vi "VI PMA Konfig.vi"() -> ()   [LabVIEW 2020, in "ABB-EL3000.lvlib" / "PMA.lvlib"]
uses:
  PMA.lvlib
  Visualisierungs Elemente/Zahlen-Ausgabefeld.ctl
  CalGas Aufschaltung/Aufschaltung CalGas_ANZEIGE.ctl
  Visualisierungs Elemente/Auswahlfeld.ctl
  FT-IR/FGV FT-IR Gasliste Aktionen.ctl
  Aktion PMA Daten allgemein.ctl
  CalGas Aufschaltung/FGV CalGas Aktionen.ctl
  Messdaten/Aktionen FGV Messdaten.ctl
  Aktion FGV Messwerte.ctl
  Passwortverwaltung/FGV Passwort Aktion.ctl
  Analysator Definition/FGV Analysator Definition Aktionen.ctl
  Kalibrieren/Kalibrierung O2.ctl
  FT-IR/FGV FT-IR Parameter.vi
  Messdaten/Messdaten.lvlib
  Passwortverwaltung/Passwort.lvlib
  Analysator Definition/Analysator Definition.lvlib
  FT-IR/FT-IR.lvlib
  Allgemein/allgemeine Sub-VIs.lvlib
  Allgemeine VI/Allgemeine VI.lvlib
  Kalibrieren/Kalibrieren.lvlib
  Allgemeine VI/Aktionen Cal Daten speichern.ctl
  CalGas Aufschaltung/CalGas Aufschaltung.lvlib
  Grafik/Grafik.lvlib
panel:
  out "Kal. Wert O2:":T1 caption="Konzentration" format="%.3f"
  out "Roh Wert O2:":sgl format="%.3f"
  in  "Kalidaten":bool
  in  "Calibration with Ambient Air:":bool
  in  "Automatic Concentration:":sgl caption="%" format="%#_5g"
  in  "Manuel Concentration:":sgl caption="%" format="%#_5g"
  in  "Calibration Mode:":enum16{"Manuel", "Automatic"}(ring)
  in  "Endpunkt":bool
  in  "0-Punkt":bool
  in  "O2 Messbereich":u16(ring)
  out "Wartungsbedarf":bool
  out "Funktionskontrolle":bool
  out "Ausfall":bool
  out "Druck Detektor:":sgl format="%#.1f"
  out "Temperatur Regler:":sgl format="%#.1f"
  out "Stellgröße Regler":sgl caption="%" format="%#.1f"
  out "Temperatur Detektor:":sgl format="%#.1f"
  out "Mwert":sgl format="%.3f"
  out "PMwert":sgl format="%.3f"
  out "O2":string
  out "Wert":T1 caption="Konzentration" format="%.3f"
  out "Graph1":waveform(dbl)[](graph)
  in  "Aufschaltung CalGas":T2 {"Aufschaltpunkt" items=["Filterblock", "Analysator direkt", "PNS", "Entnahme", "Gasdivider"]; "Kalibriergas" items=["Stickstoff"]}
  # "Konfiguration PMD"
  # "PMD"
  # "Hilfsgrößen:"
  # "Temperatur:"
  # "Stellgröße:"
  # "°C"
  # "°C"
  # "Druck:"
  # "hPa"
  # "STATUS"
  # "Aufschaltung Kalibriergas"
  # "Kalibriergas"
  # "Aufschaltpunkt"
  # "Analysator"
  # "Calibration Parameters"
  # "%"
  # "%"
  # "±"
  # "x"
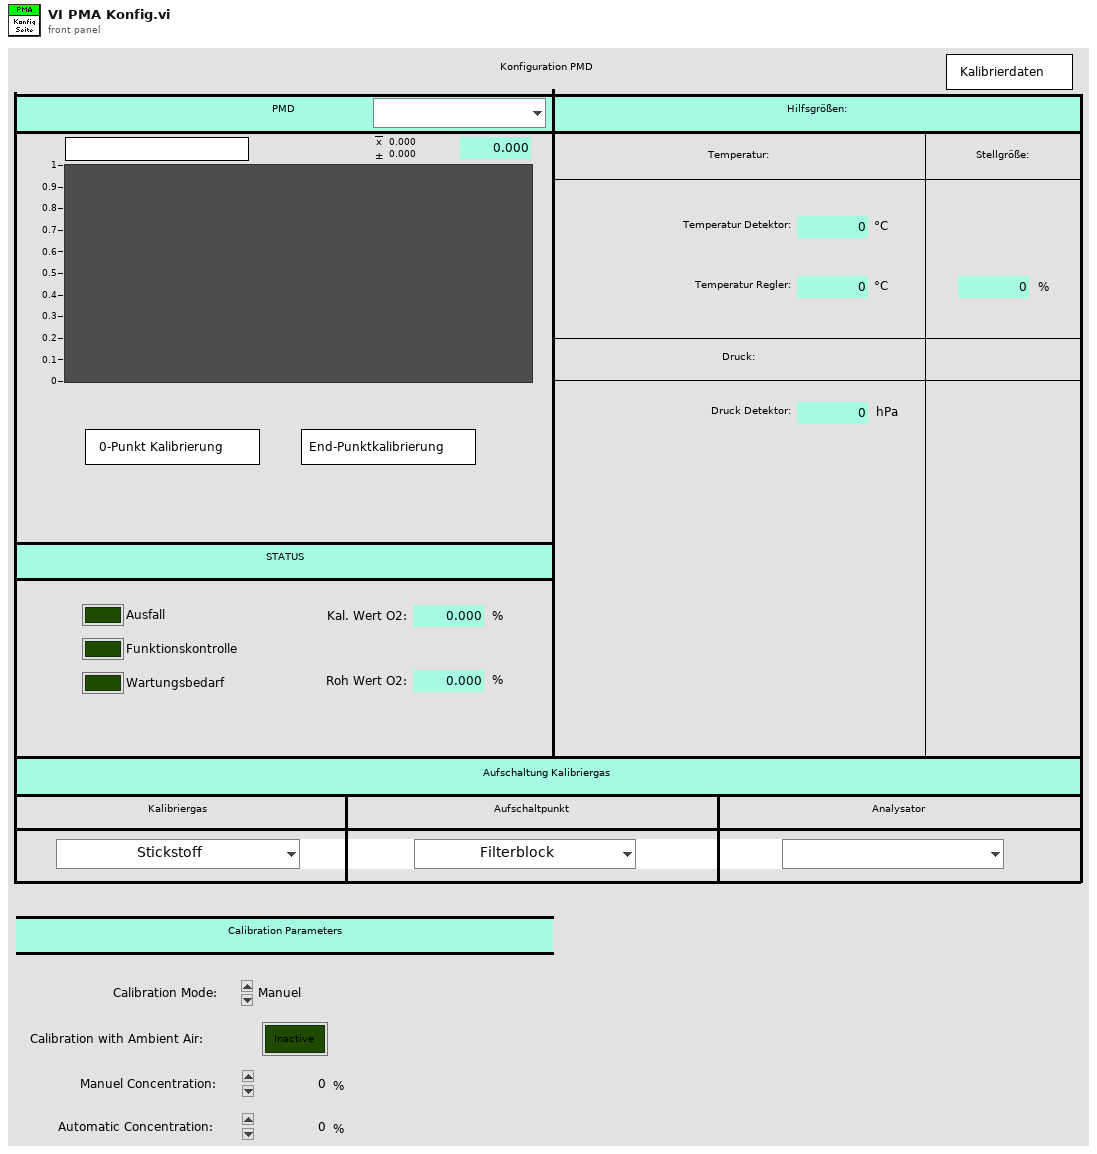
[diagram p1: front panel]
types:
  T1 = typedef "Zahlen-Ausgabefeld.ctl" = sgl
  T2 = typedef "CalGas Aufschaltung.lvlib/Aufschaltung CalGas_ANZEIGE.ctl" = cluster{"Kalibriergas":T3, "Aufschaltpunkt":T3, "Analysator":T3}
  T3 = typedef "Auswahlfeld.ctl" = u16
  T4 = typedef "CalGas Aufschaltung.lvlib/FGV CalGas Aktionen.ctl" = enum16{"lesen", "Analysator Auswahl", "Def.CalGas", "Aufschaltung CalGas", "laden", "speichern", "KAL extrahieren"}
  T5 = typedef "ABB-EL3000.lvlib/PMA.lvlib/Aktion PMA Daten allgemein.ctl" = enum16{"lesen", "schreiben", "laden ", "speichern"}
  T6 = typedef "FT-IR.lvlib/FGV FT-IR Gasliste Aktionen.ctl" = enum16{"lesen", "Gasliste FT-IR", "Gasliste ausgelesen", "laden", "speichern", "löschen"}
  T7 = typedef "ABB-EL3000.lvlib/PMA.lvlib/PMA Daten allgemein.ctl" = cluster{"Autokal aktiv":enum16{"Manuel", "Automatic"}, "Umgebungsluft Kalibration":bool}
  T8 = typedef "String - Ausgabefeld.ctl" = string
  T9 = typedef "CalGas Aufschaltung.lvlib/Aufschaltung CalGas.ctl" = cluster{"Kalibriergas":T3, "Aufschaltpunkt":T10, "Analysator":T11}
  T10 = typedef "CalGas Aufschaltung.lvlib/Auswahl Aufschaltpunkt.ctl" = enum16{"über Filterblock", "Analysator direkt", "über PNS", "Entnahme", "Gasdivider"}
  T11 = typedef "CalGas Aufschaltung.lvlib/Auswahl Analysator.ctl" = enum16{"FT-IR", "FID", "PMA", "PMA/FID/FT-IR"}
  T12 = typedef "CalGas Aufschaltung.lvlib/Definition CalGas Anzeige.ctl" = cluster{"Namen":T13, "Werte":T15, "Werte 2":T15, "Einheit":T17, "Messbereiche":T18}
  T13 = typedef "CalGas Aufschaltung.lvlib/CalGas-Namen.ctl" = cluster{"Name":T14, "Name 2":T14, "Name 3":T14, "Name 4":T14, "Name 5":T14, "Name 6":T14, "Name 7":T14, "Name 8":T14, "Name 9":T14, "Name 10":T14, "Name 11":T14, "Name 12":T14}
  T14 = typedef "String - Eingabefeld.ctl" = string
  T15 = typedef "CalGas Aufschaltung.lvlib/CalGas-Werte.ctl" = cluster{"Konzentration 1":T16, "Konzentration 2":T16, "Konzentration 3":T16, "Konzentration 4":T16, "Konzentration 5":T16, "Konzentration 6":T16, "Konzentration 7":T16, "Konzentration 8":T16, "Konzentration 9":T16, "Konzentration 10":T16, "Konzentration 11":T16, "Konzentration 12":T16}
  T16 = typedef "Zahlen-Eingabefeld.ctl" = sgl
  T17 = typedef "CalGas Aufschaltung.lvlib/CalGas-Einheit.ctl" = cluster{"Einheit 1":T3, "Einheit 2":T3, "Einheit 3":T3, "Einheit 4":T3, "Einheit 5":T3, "Einheit 6":T3, "Einheit 7":T3, "Einheit 8":T3, "Einheit 9":T3, "Einheit 10":T3, "Einheit 11":T3, "Einheit 12":T3}
  T18 = typedef "CalGas Aufschaltung.lvlib/CalGas-Messbereiche.ctl" = cluster{"Messbereich 1":T3, "Messbereich 2":T3, "Messbereich 3":T3, "Messbereich 4":T3, "Messbereich 5":T3, "Messbereich 6":T3, "Messbereich 7":T3, "Messbereich 8":T3, "Messbereich 9":T3, "Messbereich 10":T3, "Messbereich 11":T3, "Messbereich 12":T3}
  T19 = typedef "ABB-EL3000.lvlib/PMA.lvlib/Aktion FGV Messwerte.ctl" = enum16{"lesen", "Messwerte", "Messbereich", "Status", "Diagnose Werte"}
  T20 = typedef "Messdaten.lvlib/Aktionen FGV Messdaten.ctl" = enum16{"lesen", "schreiben", "löschen", "Mittelwerte", "Komponente"}
  T21 = typedef "ABB-EL3000.lvlib/Allgemeine VI.lvlib/Aktionen Cal Daten speichern.ctl" = enum16{"Cal Daten", "Toleranzen", "PMA", "FID", "Cal Daten PMA", "Cal Daten FID"}
  T22 = typedef "Passwort.lvlib/FGV Passwort Aktion.ctl" = enum16{"prüfen", "setzen", "Initialisieren", "PW speichern", "lesen", "PW Änderung"}
  T23 = typedef "Analysator Definition.lvlib/FGV Analysator Definition Aktionen.ctl" = enum16{"lesen", "MB setzen", "MB KAL setzen", "laden"}
  T24 = typedef "ABB-EL3000.lvlib/PMA.lvlib/Kalibrieren.lvlib/Kalibrierung O2.ctl" = enum16{"Nullpunkt O2", "Endpunkt O2"}
  T25 = cluster{"Temp. Detektor":sgl, "Temp. Regler":sgl, "STG Regler":sgl, "Druck Detektor":sgl}
  T26 = cluster{"Ausfall":bool, "Funktionskontrolle":bool, "Wartungsbedarf":bool}
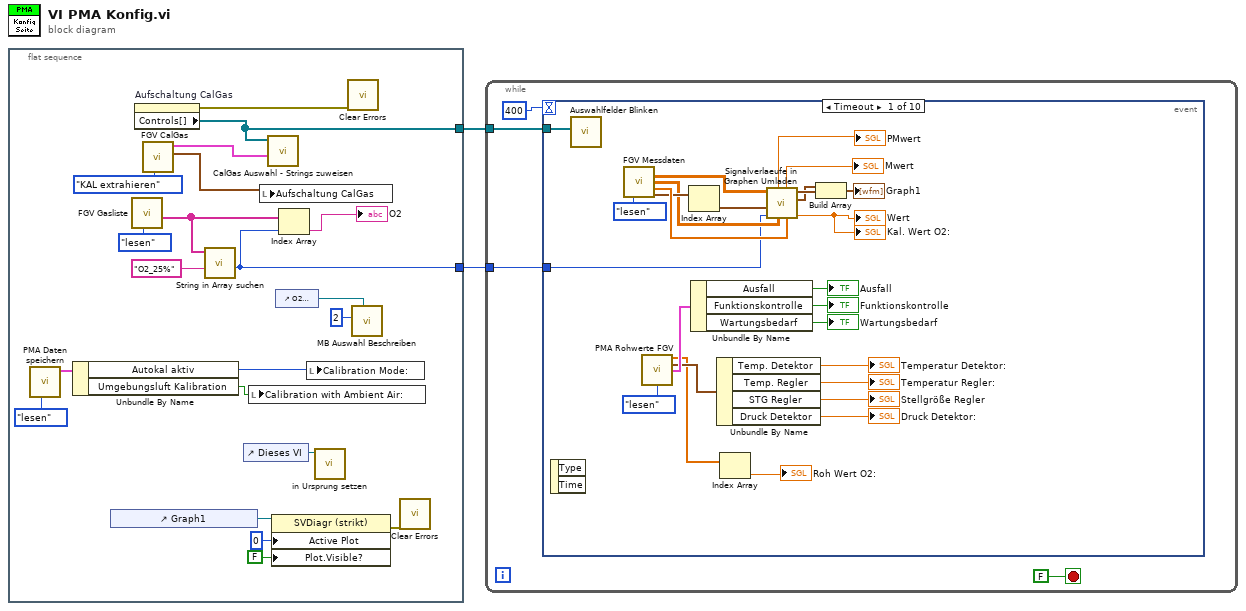
[diagram p0: block diagram]
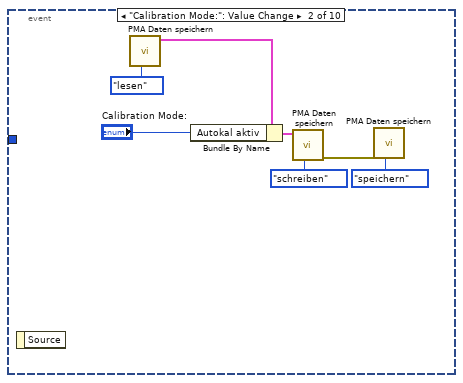
[diagram p2: hidden frame]
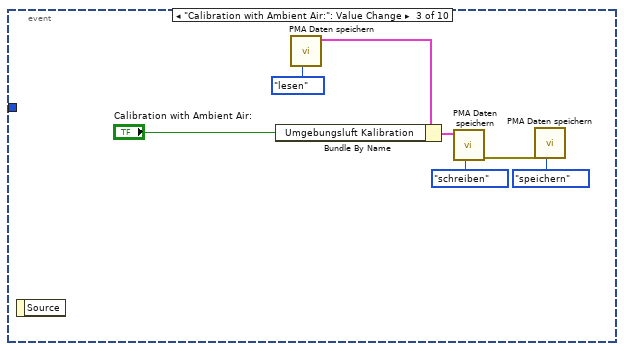
[diagram p3: hidden frame]
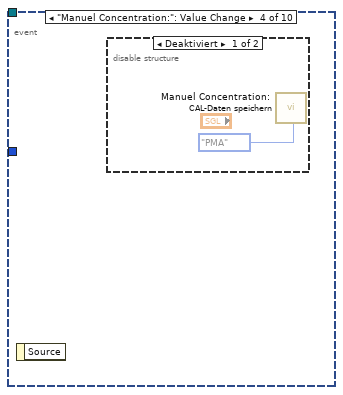
[diagram p4: hidden frame]
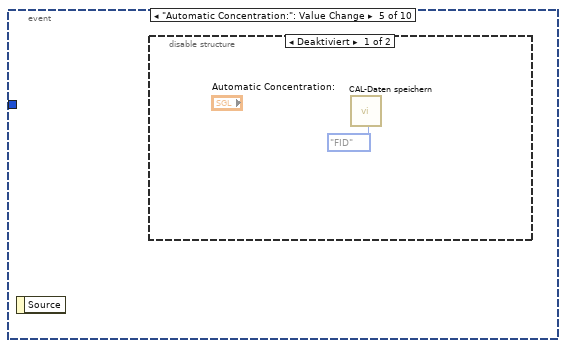
[diagram p6: hidden frame]
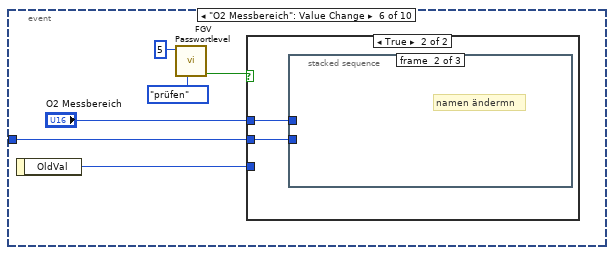
[diagram p8: hidden frame]
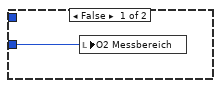
[diagram p9: hidden frame]
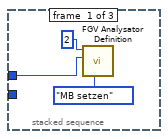
[diagram p10: hidden frame]
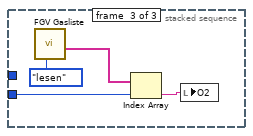
[diagram p11: hidden frame]
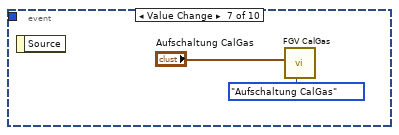
[diagram p12: hidden frame]
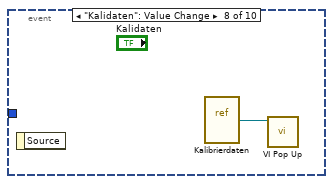
[diagram p13: hidden frame]
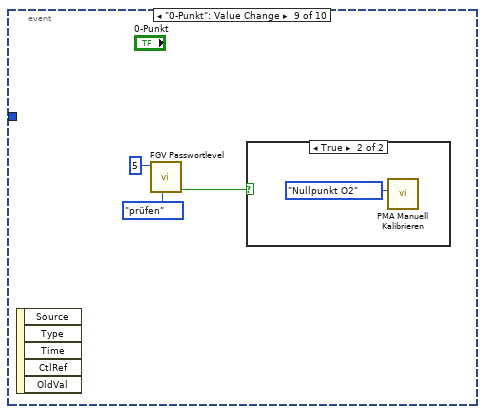
[diagram p14: hidden frame]
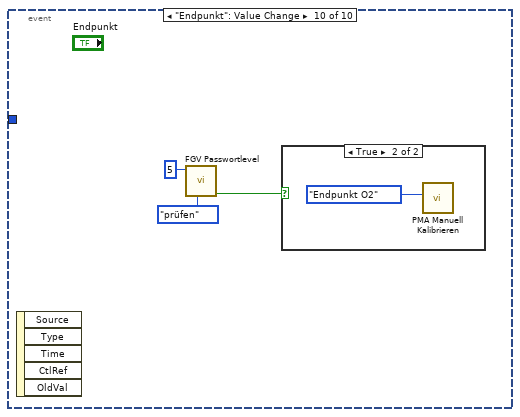
[diagram p16: hidden frame]
diagram:
  n1 = flat-sequence {
    tunnel: [w19] -> w2
    tunnel: [w3] -> w1
    frame #0 {
      n2 = call "PMA Daten speichern.vi"("Aktion"=Aktion_PMA_Daten_allgemein."lesen") -> ("PMA Daten allgemein"=w10:T7)  [unwired: 9 in, 1 out]
      n3 = Unbundle By Name(w10) -> ("Autokal aktiv"=w9:enum16{"Manuel", "Automatic"}, "Umgebungsluft Kalibration"=w8:bool)
      n4 = control-ref of="Graph1"() -> (w15:refnum<vi>)
      n5 = call "FGV Gasliste.vi"("Aktionen"=FGV_FT-IR_Gasliste_Aktionen."lesen") -> ("Aktuelle Gasliste gesamt"=w21:T8[])  [unwired: 8 in, 2 out]
      n6 = property on="Aufschaltung CalGas" class="Cluster (strikt)"() -> (error out=w4:errorcluster, "Controls[]"=w3:refnum<vi>[])  [unwired: 2 in, 1 out]
      n7 = call "FGV CalGas.vi"("Aktionen"=FGV_CalGas_Aktionen."KAL extrahieren") -> ("Aufschaltung CalGas"=w6:T9, "Def.CalGas"=w5:T12)  [unwired: 6 in, 3 out]
      n8 = call "String in Array suchen.vi"("Nach String/Zeichen suchen (-)"="O2_25%" ("DataSocket:URL"), "String-Array"=w21) -> ("Index"=w19:i32)  [unwired: 7 in, 2 out]
      n9 = control-ref of="Dieses VI"() -> (w20:refnum<vi>)
      n10 = local write "Calibration with Ambient Air:"(w8) -> ()
      n11 = local write "Aufschaltung CalGas"(w6) -> ()
      n12 = call "CalGas Auswahl - Strings zuweisen.vi"("Def.CalGas"=w5, "Aufschaltung CalGas"=w3) -> ()  [unwired: 9 in, 1 out]
      n13 = property class="SVDiagr (strikt)"(reference=w15, "Active Plot"=u32 0 ("Aktiver Plot"), "Plot.Visible?"=FALSE ("Plot.Sichtbar")) -> (error out=w12:errorcluster)  [unwired: 1 in, 1 out]
      n14 = control-ref of="O2 Messbereich"() -> (w17:refnum<vi>)
      n15 = Index Array(array=w21, index=w19) -> (element=→"O2":T8)
      n16 = local write "Calibration Mode:"(w9) -> ()
      n17 = call "in Ursprung setzen.vi"("VI Referenz"=w20) -> ()  [unwired: 10 in, 1 out]
      n18 = call <vilib>:"Clear Errors.vi"("error in (no error)"=w4) -> ()  [unwired: 5 in, 2 out]
      n19 = call "MB Auswahl Beschreiben.vi"("Auswahl Referenz"=w17, "Komponente"=2) -> ()  [unwired: 10 in]
      n20 = call <vilib>:"Clear Errors.vi"("error in (no error)"=w12) -> ()  [unwired: 5 in, 2 out]
    }
  }
  n21 = while {
    tunnel: w2 -> [w25]
    tunnel: w1 -> [w24]
    stop <- FALSE stop-if-true
    n22 = event shown="[0] Timeout" {
      selector: _ -> [_ _ _ _ _ _ _ _ _ _]
      dyn-events: _ -> [_ _ _ _ _ _ _ _ _ _]
      timeout: 400 -> [_ _ _ _ _ _ _ _ _ _]
      tunnel: w25 -> [w36 _ _ _ _ w71 _ _ _ _]
      tunnel: w24 -> [w30 _ _ _ _ _ _ _ _ _]
      event Timeout {
        n23 = event-data() -> ()  [unwired: 1 in, 2 out]
        n24 = call "Auswahlfelder Blinken.vi"("Controls[]"=w30) -> ()  [unwired: 11 in]
        n25 = call "FGV Messdaten.vi"("Aktionen"=Aktionen_FGV_Messdaten."lesen") -> ("Messdaten"=w49:sgl[][], "Mittelwertdaten"=w48:sgl[][], "Deviation"=w53:sgl[], "Zeitstempeln"=w51:timestamp[])  [unwired: 6 in, 5 out]
        n26 = call "PMA Rohwerte FGV.vi"("Aktion"=Aktion_FGV_Messwerte."lesen") -> ("Messwerte"=w32:sgl[], "Diagnose Werte"=w40:T25, "Status"=w44:T26)  [unwired: 11 in, 1 out]
        n27 = Index Array(array=w51) -> (element=w52:timestamp)  [unwired: 1 in]
        n28 = Unbundle By Name(w44) -> ("Ausfall"=→"Ausfall":bool, "Funktionskontrolle"=→"Funktionskontrolle":bool, "Wartungsbedarf"=→"Wartungsbedarf":bool)
        n29 = Unbundle By Name(w40) -> ("Temp. Detektor"=→"Temperatur Detektor:":sgl, "Temp. Regler"=→"Temperatur Regler:":sgl, "STG Regler"=→"Stellgröße Regler":sgl, "Druck Detektor"=→"Druck Detektor:":sgl)
        n30 = Index Array(array=w32) -> (element=→"Roh Wert O2:":sgl)  [unwired: 1 in]
        n31 = call "Signalverlaeufe in Graphen Umladen.vi"("Deviation"=w53, "Mittelwertdaten"=w48, "Gas-Auswahl"=w36, "t0"=w52, "Werte"=w49) -> ("Konzentration"=→"Wert" →"Kal. Wert O2:":sgl, "Mittelwert"=w34:waveform(dbl), "Waveform"=w35:waveform(dbl), "aktuelle Mittelwert"=→"Mwert":sgl, "Deviation"=→"PMwert":sgl)  [unwired: 2 in]
        n32 = Build Array(w34, w35) -> (→"Graph1":waveform(dbl)[])
      }
      event "Calibration Mode:": Value Change {
        n33 = event-data() -> ()  [unwired: 1 in, 1 out]
        n34 = call "PMA Daten speichern.vi"("Aktion"=Aktion_PMA_Daten_allgemein."lesen") -> ("PMA Daten allgemein"=w56:T7)  [unwired: 9 in, 1 out]
        n35 = Bundle By Name(cluster=w56, "Autokal aktiv"="Calibration Mode:") -> (w55:T7)
        n36 = call "PMA Daten speichern.vi"("Aktion"=Aktion_PMA_Daten_allgemein."schreiben", "PMA Daten allgemein"=w55) -> ("error out"=w58:errorcluster)  [unwired: 8 in, 1 out]
        n37 = call "PMA Daten speichern.vi"("Aktion"=Aktion_PMA_Daten_allgemein."speichern", "error in (no error)"=w58) -> ()  [unwired: 8 in, 2 out]
      }
      event "Calibration with Ambient Air:": Value Change {
        n38 = event-data() -> ()  [unwired: 1 in, 1 out]
        n39 = call "PMA Daten speichern.vi"("Aktion"=Aktion_PMA_Daten_allgemein."lesen") -> ("PMA Daten allgemein"=w63:T7)  [unwired: 9 in, 1 out]
        n40 = Bundle By Name(cluster=w63, "Umgebungsluft Kalibration"="Calibration with Ambient Air:") -> (w62:T7)
        n41 = call "PMA Daten speichern.vi"("Aktion"=Aktion_PMA_Daten_allgemein."schreiben", "PMA Daten allgemein"=w62) -> ("error out"=w65:errorcluster)  [unwired: 8 in, 1 out]
        n42 = call "PMA Daten speichern.vi"("Aktion"=Aktion_PMA_Daten_allgemein."speichern", "error in (no error)"=w65) -> ()  [unwired: 8 in, 2 out]
      }
      event "Manuel Concentration:": Value Change {
        n43 = event-data() -> ()  [unwired: 1 in, 1 out]
        n44 = disable-structure shown="Deaktiviert" {
          frame Disabled {
            n45 = call "CAL-Daten speichern.vi"("Aktionen Kal Daten speichern"=Aktionen_Cal_Daten_speichern."PMA") -> ()  [unwired: 19 in]
          }
          frame Enabled {
          }
        }
      }
      event "Automatic Concentration:": Value Change {
        n46 = event-data() -> ()  [unwired: 1 in, 1 out]
        n47 = disable-structure shown="Deaktiviert" {
          frame Disabled {
            n48 = call "CAL-Daten speichern.vi"("Aktionen Kal Daten speichern"=Aktionen_Cal_Daten_speichern."FID") -> ()  [unwired: 19 in]
          }
          frame Enabled {
          }
        }
      }
      event "O2 Messbereich": Value Change {
        n49 = event-data() -> ("OldVal"=w72:u16)  [unwired: 1 in]
        n50 = call "FGV Passwortlevel.vi"("FGV Passwort Aktion"=FGV_Passwort_Aktion."prüfen", "geforderter Level"=i16 5) -> ("Freigabe"=w73:bool)  [unwired: 7 in, 2 out]
        n51 = case shown="True" w73 {
          tunnel: w72 -> [w76 _]
          tunnel: w71 -> [_ w78]
          tunnel: "O2 Messbereich" -> [_ w77]
          frame False {
            n52 = local write "O2 Messbereich"(w76) -> ()
          }
          frame True {
            n53 = stacked-sequence {
              tunnel: w78 -> [_ _ w83]
              tunnel: w77 -> [w79 _ _]
              frame #0 {
                n54 = call "FGV Analysator Definition.vi"("Aktionen"=FGV_Analysator_Definition_Aktionen."MB setzen", "Messbereich"=w79, "Komponente"=2) -> ()  [unwired: 4 in, 5 out]
              }
              frame #1 {
                # "namen ändermn"
              }
              frame #2 {
                n55 = call "FGV Gasliste.vi"("Aktionen"=FGV_FT-IR_Gasliste_Aktionen."lesen") -> ("Aktuelle Gasliste gesamt"=w85:T8[])  [unwired: 8 in, 2 out]
                n56 = Index Array(array=w85, index=w83) -> (element=w82:T8)
                n57 = local write "O2"(w82) -> ()
              }
            }
          }
        }
      }
      event Value Change {
        n58 = event-data() -> ()  [unwired: 1 in, 1 out]
        n59 = call "FGV CalGas.vi"("Aktionen"=FGV_CalGas_Aktionen."Aufschaltung CalGas", "Aufschaltung CalGas"="Aufschaltung CalGas") -> ()  [unwired: 5 in, 5 out]
      }
      event "Kalidaten": Value Change {
        n60 = event-data() -> ()  [unwired: 1 in, 1 out]
        n61 = vi-ref "Kalibrierdaten.vi"() -> (w88:refnum<vi>)
        n62 = call "VI Pop Up.vi"("VI Referenz"=w88) -> ()  [unwired: 10 in, 1 out]
      }
      event "0-Punkt": Value Change {
        n63 = event-data() -> ()  [unwired: 1 in, 5 out]
        n64 = call "FGV Passwortlevel.vi"("FGV Passwort Aktion"=FGV_Passwort_Aktion."prüfen", "geforderter Level"=i16 5) -> ("Freigabe"=w89:bool)  [unwired: 7 in, 2 out]
        n65 = case shown="True" w89 {
          frame False {
          }
          frame True {
            n66 = call "PMA Manuell Kalibrieren.vi"("Kalibrieren"=Kalibrierung_O2."Nullpunkt O2") -> ()  [unwired: 9 in, 2 out]
          }
        }
      }
      event "Endpunkt": Value Change {
        n67 = event-data() -> ()  [unwired: 1 in, 5 out]
        n68 = call "FGV Passwortlevel.vi"("FGV Passwort Aktion"=FGV_Passwort_Aktion."prüfen", "geforderter Level"=i16 5) -> ("Freigabe"=w93:bool)  [unwired: 7 in, 2 out]
        n69 = case shown="True" w93 {
          frame False {
          }
          frame True {
            n70 = call "PMA Manuell Kalibrieren.vi"("Kalibrieren"=Kalibrierung_O2."Endpunkt O2") -> ()  [unwired: 9 in, 2 out]
          }
        }
      }
    }
  }
